vi "obtain_cancel_token.vi"(8 "error in (no error)":errorcluster) -> (0 "error out":errorcluster, 3 "cancel_token":refnum<queue>)   [LabVIEW 2021, in "system.threading.lvclass"]
uses:
  system.threading.lvclass
  system.threading.lvclass/system.threading.ctl
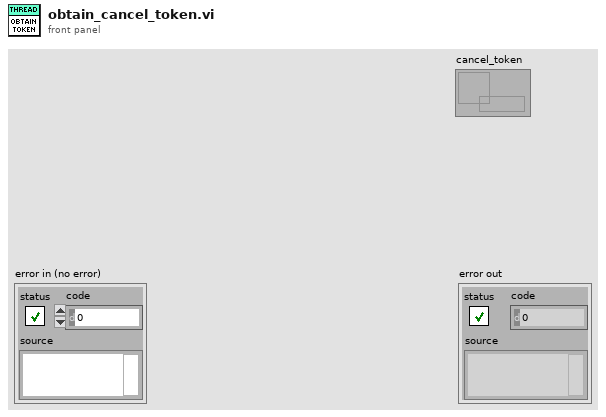
[diagram p1: front panel]
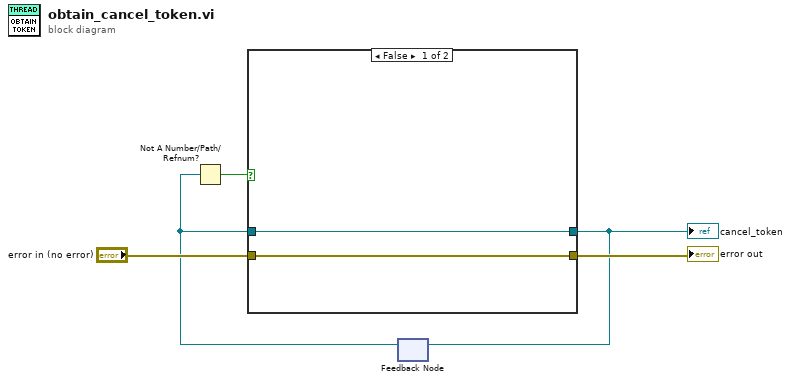
[diagram p0: block diagram]
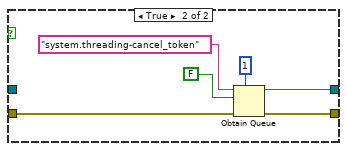
[diagram p2: hidden frame]
diagram:
  n1 = feedback #1() -> (w1:refnum<queue>)  [unwired: 1 in]
  n2 = Not A Number/Path/Refnum?(number/path/refnum=w1) -> (NaN/Path/Refnum?=w2:bool)
  n3 = case shown="False" w2 {
    tunnel: "error in (no error)" -> [w6 w13]
    tunnel: [w7 w9] -> w3
    tunnel: [w6 w8] -> w4
    tunnel: w1 -> [w7 _]
    frame False {
    }
    frame True {
      n4 = Obtain Queue(max queue size (-1, unlimited)=1, name (unnamed)="system.threading-cancel_token", element data type=FALSE, error in (no error)=w13) -> (queue out=w9:refnum<queue>, error out=w8:errorcluster)  [unwired: 1 in, 1 out]
    }
  }
  "error out" <- w4
  "cancel_token" <- w3
  n5 = feedback-in #1(w3) -> ()
